vi "ADIS16448_RoboRIO_Teensy_Loop.vi"(8 "error in":errorcluster, 11 "SerialPortRefIn":T1) -> ()   [LabVIEW 2016, in "RoboRIO-Teensy-ADIS16448-Interface.lvlib"]
uses:
  RoboRIO-Teensy-ADIS16448-Interface.lvlib
  <vilib>/Rock Robotics/WPI/SerialPort/WPI_SerialPortRef.ctl
panel:
  in  "Main Name":string
  out "Parsed Serial Data":dbl[](array[numeric])
  out "Raw Serial Data":string
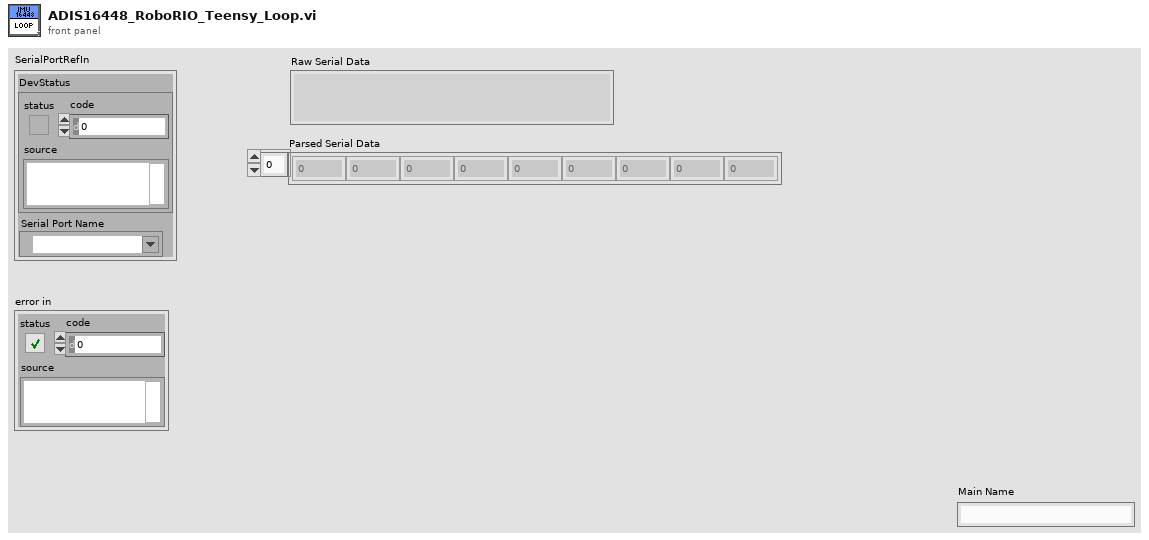
[diagram p1: front panel]
types:
  T1 = typedef "WPI_SerialPortRef.ctl" = cluster{"DevStatus":errorcluster, "Serial Port Name":refnum<visa-resource-name>}
  T2 = cluster{"X Angle":dbl, "Y Angle":dbl, "Z Angle":dbl}
  T3 = enum32{"Bad", "Idle", "Run top level", "Running"}
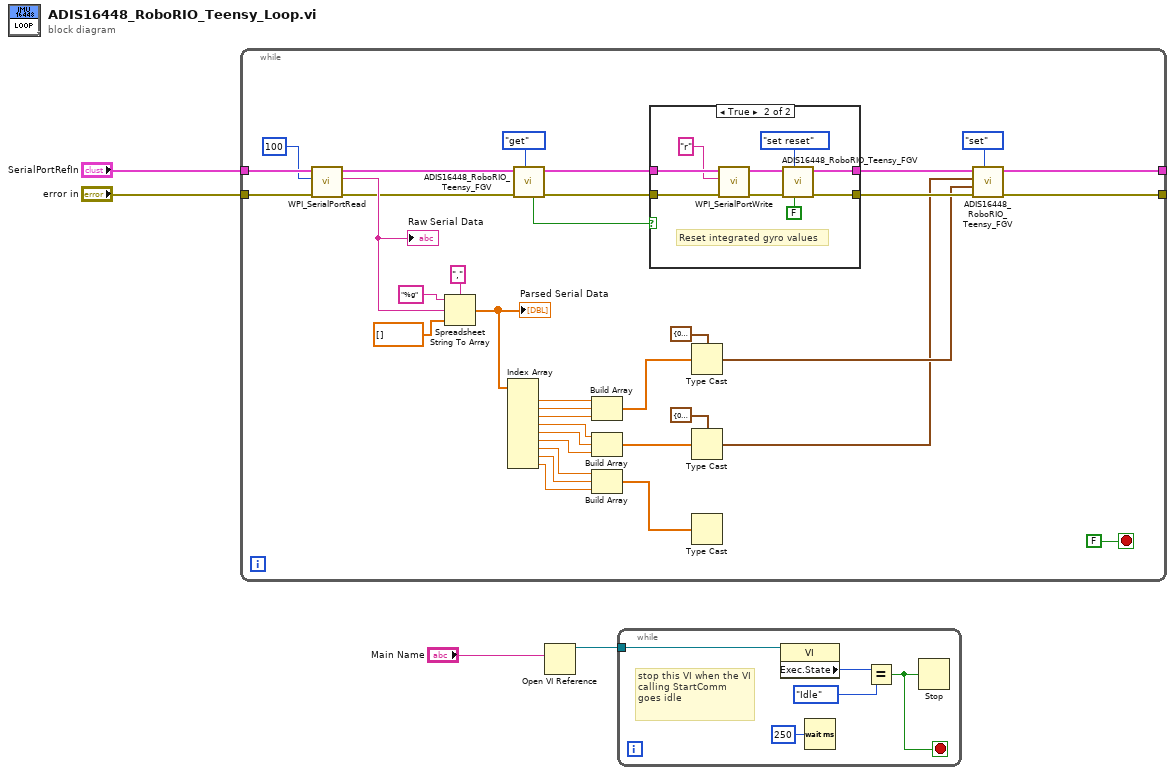
[diagram p0: block diagram]
diagram:
  n1 = while {
    tunnel: "SerialPortRefIn" -> [w40]
    tunnel: "error in" -> [w39]
    tunnel: [w24] -> _
    tunnel: [w23] -> _
    stop <- FALSE stop-if-true
    n2 = call <vilib>:"WPI_SerialPortRead.vi"("error in (no error)"=w39, "Num Bytes to Read"=u32 100, "SerialPortRef"=w40) -> ("error out"=w27:errorcluster, "Buffer"=w34:string, "SerialPortRef"=w31:T1)  [unwired: 6 in]
    "Raw Serial Data" <- w34
    n3 = Spreadsheet String To Array(delimiter (Tab)="," ("delimiter"), format string="%g", spreadsheet string=w34, array type (2D Dbl)=dbl[] []) -> (array=w21:dbl[])
    "Parsed Serial Data" <- w21
    n4 = Index Array(array=w21) -> (element #1=w20:dbl, element #2=w19:dbl, element #3=w18:dbl, element #4=w16:dbl, element #5=w15:dbl, element #6=w14:dbl, element #7=w7:dbl, element #8=w6:dbl, element #9=w8:dbl)  [unwired: 9 in]
    n5 = call "ADIS16448_RoboRIO_Teensy_FGV.vi"("Operation"=enum16{"set", "get", "set reset"}."get", "error in"=w27, "SerialPortRefIn"=w31) -> ("error out"=w28:errorcluster, "SerialPortRefOut"=w29:T1, "Reset Out"=w30:bool)  [unwired: 4 in, 2 out]
    n6 = Build Array(w20, w19, w18) -> (w17:dbl[])
    n7 = Build Array(w16, w15, w14) -> (w13:dbl[])
    n8 = Build Array(w7, w6, w8) -> (w5:dbl[])
    n9 = case shown="True" w30 {
      tunnel: w29 -> [w42 w51]
      tunnel: w28 -> [w41 w50]
      tunnel: [w42 w46] -> w26
      tunnel: [w41 w45] -> w25
      frame False {
      }
      frame True {
        # "Reset integrated gyro values"
        n10 = call <vilib>:"WPI_SerialPortWrite.vi"("error in (no error)"=w50, "Buffer"="r", "SerialPortRef"=w51) -> ("error out"=w44:errorcluster, "SerialPortRef"=w43:T1)  [unwired: 6 in, 1 out]
        n11 = call "ADIS16448_RoboRIO_Teensy_FGV.vi"("Reset"=FALSE, "Operation"=enum16{"set", "get", "set reset"}."set reset", "error in"=w44, "SerialPortRefIn"=w43) -> ("error out"=w45:errorcluster, "SerialPortRefOut"=w46:T1)  [unwired: 3 in, 3 out]
      }
    }
    n12 = Type Cast(type=cluster{"Pitch":dbl, "Roll":dbl, "Yaw":dbl} {"Pitch"=0.0, "Roll"=0.0, "Yaw"=0.0} ("IMU AHRS"), x=w17) -> (*(type *) &x=w10:cluster{"Pitch":dbl, "Roll":dbl, "Yaw":dbl})
    n13 = Type Cast(type=T2 {"X Angle"=0.0, "Y Angle"=0.0, "Z Angle"=0.0} ("IMU Angles"), x=w13) -> (*(type *) &x=w9:T2)
    n14 = Type Cast(x=w5) -> ()  [unwired: 1 in, 1 out]
    n15 = call "ADIS16448_RoboRIO_Teensy_FGV.vi"("Operation"=enum16{"set", "get", "set reset"}."set", "error in"=w25, "IMU AHRS"=w10, "IMU Angles"=w9, "SerialPortRefIn"=w26) -> ("error out"=w23:errorcluster, "SerialPortRefOut"=w24:T1)  [unwired: 2 in, 3 out]
  }
  n16 = Open VI Reference(vi path="Main Name") -> (vi reference=w2:refnum<vi>)  [unwired: 1 in, 5 out]
  n17 = while {
    tunnel: w2 -> [w53]
    stop <- w52 stop-if-true
    # "stop this VI when the VI calling StartComm goes idle"
    n18 = property class="VI"(reference=w53) -> ("Exec.State"=w55:T3)  [unwired: 1 in, 2 out]
    n19 = Wait (ms)(milliseconds to wait=u32 250) -> ()  [unwired: 1 out]
    n20 = Equal?(x=w55, y=T3."Idle" ("Execution:State")) -> (x = y?=w52:bool)
    n21 = Stop(stop? (T)=w52) -> ()
  }
